vi "XL320_Write U8 To 1 Address.vi"(0 "VISA resource name":refnum<visa-resource-name>, 5 "Motor ID (0)":u8, 7 "Address number (0)":u16, 9 "Parameter (0)":u8, 11 "error in (no error)":errorcluster) -> (4 "VISA resource name out":refnum<visa-resource-name>, 15 "error out":errorcluster)   [LabVIEW 2017, in "Dynamixel XL320.lvlib"]
doc: "Writes a U8 to one address of the register on the motor. This is a Low-Level VI that is used by other VIs."
uses:
  <instrlib>/Dynamixel XL320 (Drivers instrument)/Dynamixel XL320.lvlib
  <instrlib>/Dynamixel XL320 (Drivers instrument)/Public/Configure/XL320_Select_Action.ctl
panel:
  # "Ghislain REMY, IUT de Cachan, 2015 December 2015"
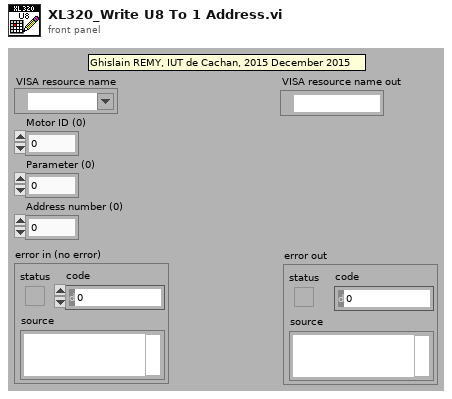
[diagram p1: front panel]
types:
  T1 = typedef "Dynamixel XL320.lvlib/XL320_Select_Action.ctl" = u8
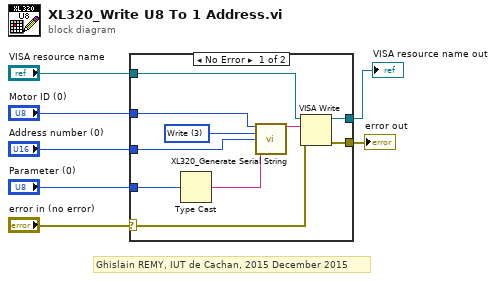
[diagram p0: block diagram]
diagram:
  # "Ghislain REMY, IUT de Cachan, 2015 December 2015"
  n1 = case shown="No Error" "error in (no error)" {
    selector: "error in (no error)" -> [w14 w19]
    tunnel: "Parameter (0)" -> [w13 _]
    tunnel: "Address number (0)" -> [w9 _]
    tunnel: "Motor ID (0)" -> [w10 _]
    tunnel: "VISA resource name" -> [w17 w18]
    tunnel: [w16 w19] -> w3
    tunnel: [w15 w18] -> w2
    frame No Error {
      w8 = T1 3 items=["Ping"=1, "Read"=2, "Write"=3, "Registered Write"=4, "Action"=5, "Reset"=6, "Reboot"=8, "Status"=85, "Sync Read"=130, "Sync Write"=131, "Bulk Read"=146, "Bulk Write"=147] ("Select Action")
      n2 = Type Cast(x=w13) -> (*(type *) &x=w11:string)  [unwired: 1 in]
      n3 = call <instrlib>:"XL320_Generate Serial String.vi"("Motor ID"=w10, "Select Action"=w8, "Address"=w9, "Parameters"=w11) -> ("Command to Serial"=w12:string)  [unwired: 10 in, 1 out]
      n4 = VISA Write(VISA resource name=w17, write buffer=w12, error in (no error)=w14) -> (VISA resource name out=w15:refnum<visa-resource-name>, error out=w16:errorcluster)  [unwired: 1 out]
    }
    frame Error {
    }
  }
  "error out" <- w3
  "VISA resource name out" <- w2
